vi "Convert Loader Type to gRPC Type.vi"(11 "Loader Type":T2) -> (3 "Loader Type":T1)   [LabVIEW 2021, in "CIFPluginManager.lvclass"]
uses:
  CIFPluginManager.lvclass
  CIFPluginManager.lvclass/CIFPluginManager.ctl
  gRPC/CIF_Manager_server/RPC Messages/cif_manager_LoaderType.ctl
  gRPC/CIF_Manager_server/CIF_Manager_server.lvlib
  typedef/Loader Type.ctl
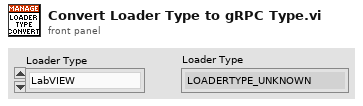
[diagram p1: front panel]
types:
  T1 = typedef "CIF_Manager_server.lvlib/cif_manager_LoaderType.ctl" = enum32{"LOADERTYPE_UNKNOWN", "LOADERTYPE_LABVIEW"}
  T2 = typedef "CIFPluginManager.lvclass/Loader Type.ctl" = enum16{"LabVIEW"}
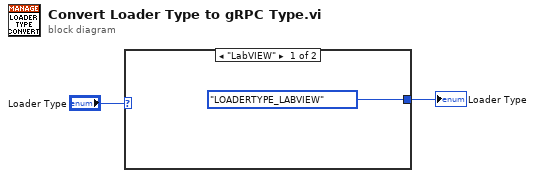
[diagram p0: block diagram]
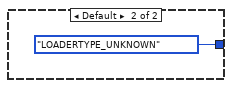
[diagram p2: hidden frame]
diagram:
  n1 = case shown="\"LabVIEW\"" "Loader Type" {
    tunnel: [cif_manager_LoaderType."LOADERTYPE_LABVIEW" ("launcher_type") cif_manager_LoaderType."LOADERTYPE_UNKNOWN" ("launcher_type")] -> w1
    frame "LabVIEW" {
    }
    frame Default {
    }
  }
  "Loader Type" <- w1
